vi "DAQ.Stop.vi"(8 "error in (no error)":errorcluster, 11 "Instrument.DAQ in":refnum<class "Instrument.DAQ.lvclass">) -> (0 "error out":errorcluster, 3 "Instrument.DAQ out":refnum<class "Instrument.DAQ.lvclass">)   [LabVIEW 2019, in "Instrument.Lockin.lvlib" / "Instrument.DAQ.lvclass"]
uses:
  Instrument.DAQ.lvclass
  DAQmx/typedefs/DAQmx.Commands--enum.ctl
  Instrument.DAQ.lvclass/Instrument.DAQ.ctl
  DAQmx/DAQmx.lvclass
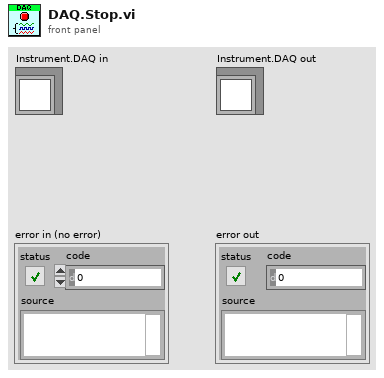
[diagram p1: front panel]
types:
  T1 = typedef "DAQmx.lvclass/DAQmx.Commands--enum.ctl" = enum16{"idle", "start", "stop", "calibrate", "auto", "exit"}
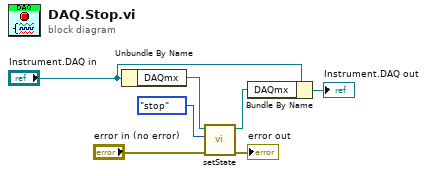
[diagram p0: block diagram]
diagram:
  n1 = Unbundle By Name("Instrument.DAQ in") -> ("DAQmx"=w5:refnum<class "DAQmx.lvclass">)
  n2 = call "setState.vi"("error in (no error)"="error in (no error)", "Command"=DAQmx.Commands--enum."stop" ("State"), "DAQmx in"=w5) -> ("error out"=→"error out":errorcluster, "DAQmx out"=w4:refnum<class "DAQmx.lvclass">)  [unwired: 7 in]
  n3 = Bundle By Name(cluster="Instrument.DAQ in", "DAQmx"=w4) -> (→"Instrument.DAQ out":refnum<class "Instrument.DAQ.lvclass">)
